vi "Status changed.vi"(1 "Overall status 2":T1={"Desired"={"Field [T]"=0.0, "Ramp [T/s]"=0.0, "Custom Ramp?"=TRUE, "Mode"=enum."Ramping"}, "Actual"={"Mode"=enum."Persistant", "Ramping output"=enum."At Target", "Ready for change"=FALSE, "Switch heater"=FALSE, "Cooler Overheat"=FALSE, "Coil overheat"=FALSE, "Energized"=FALSE, "Output [T]"=0.0, "Field [T]"=0.0, "Ramp[T/s]"=0.0, "Switch\ntemperature [K]"=0.0, "Voltage [V]"=0.0, "Current direction"=FALSE}}, 2 "Overall status":T1={"Desired"={"Field [T]"=0.0, "Ramp [T/s]"=0.0, "Custom Ramp?"=TRUE, "Mode"=enum."Ramping"}, "Actual"={"Mode"=enum."Persistant", "Ramping output"=enum."At Target", "Ready for change"=FALSE, "Switch heater"=FALSE, "Cooler Overheat"=FALSE, "Coil overheat"=FALSE, "Energized"=FALSE, "Output [T]"=0.0, "Field [T]"=0.0, "Ramp[T/s]"=0.0, "Switch\ntemperature [K]"=0.0, "Voltage [V]"=0.0, "Current direction"=FALSE}}) -> (0 "Changed":bool)   [LabVIEW 2024, in "Magnet module.lvlib"]
uses:
  Magnet module.lvlib
  ctl/RampingOutput.ctl
  ctl/Magnet mode.ctl
  ctl/SetField data.ctl
  ctl/Overall status.ctl
  ctl/Magnet mode public.ctl
  ctl/Actual magnet state.ctl
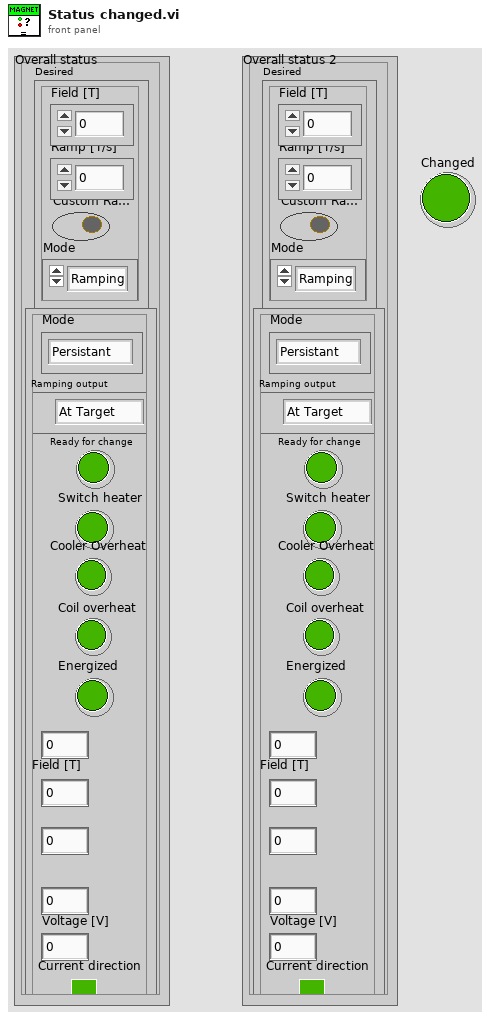
[diagram p1: front panel]
types:
  T1 = typedef "Magnet module.lvlib/Overall status.ctl" = cluster{"Desired":T2, "Actual":T4}
  T2 = typedef "Magnet module.lvlib/SetField data.ctl" = cluster{"Field [T]":dbl, "Ramp [T/s]":dbl, "Custom Ramp?":bool, "Mode":T3}
  T3 = typedef "Magnet module.lvlib/Magnet mode public.ctl" = enum16{"Persistant", "Ramping"}
  T4 = typedef "Magnet module.lvlib/Actual magnet state.ctl" = cluster{"Mode":T5, "Ramping output":T6, "Ready for change":bool, "Switch heater":bool, "Cooler Overheat":bool, "Coil overheat":bool, "Energized":bool, "Output [T]":dbl, "Field [T]":dbl, "Ramp[T/s]":dbl, "Switch\ntemperature [K]":dbl, "Voltage [V]":dbl, "Current direction":bool}
  T5 = typedef "Magnet module.lvlib/Magnet mode.ctl" = enum16{"Persistant", "Switching", "Ramping", "Quenched"}
  T6 = typedef "Magnet module.lvlib/RampingOutput.ctl" = enum16{"At Target", "Go up", "Go down"}
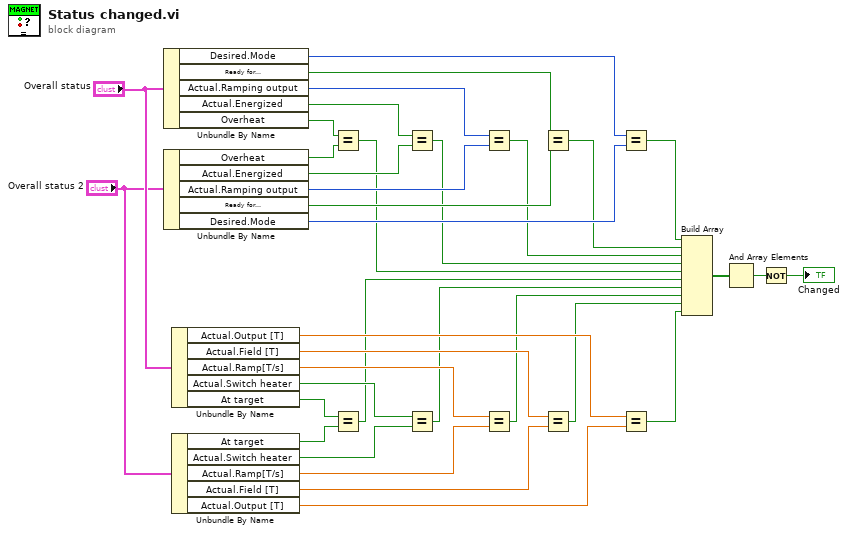
[diagram p0: block diagram]
diagram:
  n1 = Unbundle By Name("Overall status") -> ("Desired.Mode"=w23:T3, "Ready for\nmode change"=w21:bool, "Actual.Ramping output"=w19:T6, "Actual.Energized"=w17:bool, "Overheat"=w15:bool)
  n2 = Unbundle By Name("Overall status 2") -> ("Overheat"=w14:bool, "Actual.Energized"=w16:bool, "Actual.Ramping output"=w18:T6, "Ready for\nmode change"=w20:bool, "Desired.Mode"=w22:T3)
  n3 = Unbundle By Name("Overall status") -> ("Actual.Output [T]"=w33:dbl, "Actual.Field [T]"=w26:dbl, "Actual.Ramp[T/s]"=w28:dbl, "Actual.Switch heater"=w30:bool, "At target"=w32:bool)
  n4 = Unbundle By Name("Overall status 2") -> ("At target"=w31:bool, "Actual.Switch heater"=w29:bool, "Actual.Ramp[T/s]"=w27:dbl, "Actual.Field [T]"=w25:dbl, "Actual.Output [T]"=w24:dbl)
  n5 = Equal?(x=w15, y=w14) -> (x = y?=w9:bool)
  n6 = Equal?(x=w32, y=w31) -> (x = y?=w4:bool)
  n7 = Equal?(x=w17, y=w16) -> (x = y?=w10:bool)
  n8 = Equal?(x=w30, y=w29) -> (x = y?=w5:bool)
  n9 = Equal?(x=w19, y=w18) -> (x = y?=w11:bool)
  n10 = Equal?(x=w28, y=w27) -> (x = y?=w6:bool)
  n11 = Equal?(x=w21, y=w20) -> (x = y?=w12:bool)
  n12 = Equal?(x=w26, y=w25) -> (x = y?=w7:bool)
  n13 = Equal?(x=w23, y=w22) -> (x = y?=w13:bool)
  n14 = Equal?(x=w33, y=w24) -> (x = y?=w8:bool)
  n15 = Build Array(w13, w12, w11, w10, w9, w4, w5, w6, w7, w8) -> (w3:bool[])
  n16 = And Array Elements(Boolean array=w3) -> (logical AND=w2:bool)
  n17 = Not(x=w2) -> (.not. x?=→"Changed":bool)
